vi "Line to ROI.vi"(6 "error in (no error)":errorcluster, 8 "End Y":i32, 9 "End X":i32, 10 "Start Y":i32, 11 "Start X":i32) -> (0 "error out":errorcluster, 3 "ROI Descriptor":T1 {"Contours"."Type" items=["No Selection", "Point", "Line", "Rectangle", "Oval", "Polygon", "Freehand Region", "Annulus", "Unused2", "Unused3", "Broken Line", "Freehand Line", "Rotated Rectangle"]})   [LabVIEW 2016]
panel:
  # "Coordinates of the line"
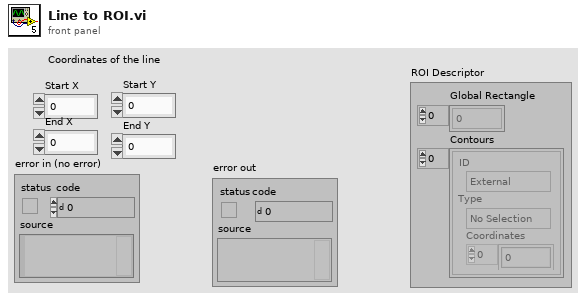
[diagram p1: front panel]
types:
  T1 = typedef "ROI Descriptor" = cluster{"Global Rectangle":i32[], "Contours":cluster{"ID":enum32{"External", "Internal"}, "Type":u32, "Coordinates":i32[]}[]}
  T2 = typedef "IMAQ Line" = cluster{"Start X":i32, "Start Y":i32, "End X":i32, "End Y":i32}
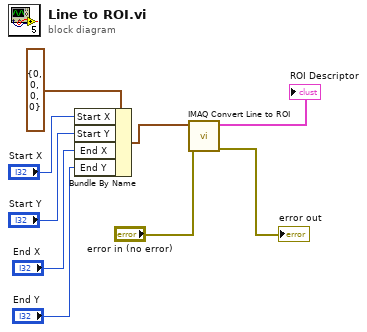
[diagram p0: block diagram]
diagram:
  n1 = Bundle By Name(cluster=T2 {"Start X"=0, "Start Y"=0, "End X"=0, "End Y"=0} ("Line"), "Start X"="Start X", "Start Y"="Start Y", "End X"="End X", "End Y"="End Y") -> (w8:T2)
  n2 = call "IMAQ Convert Line to ROI"("error in (no error)"="error in (no error)", "Line"=w8) -> ("error out"=→"error out":errorcluster, "ROI Descriptor"=→"ROI Descriptor":T1)  [unwired: 7 in]
